vi "ConvertArrayToMessages.vi"(8 "error in (no error)":errorcluster, 11 "Array":bool[][](array[boolean])=array64x128[8192 elements]) -> (0 "error out":errorcluster, 3 "Messages":string[](array[string]))   [LabVIEW 2020, in "CTI-Peripheral.lvlib" / "48x64 I2C OLED SSD1306.lvclass"]
uses:
  48x64 I2C OLED SSD1306.lvclass
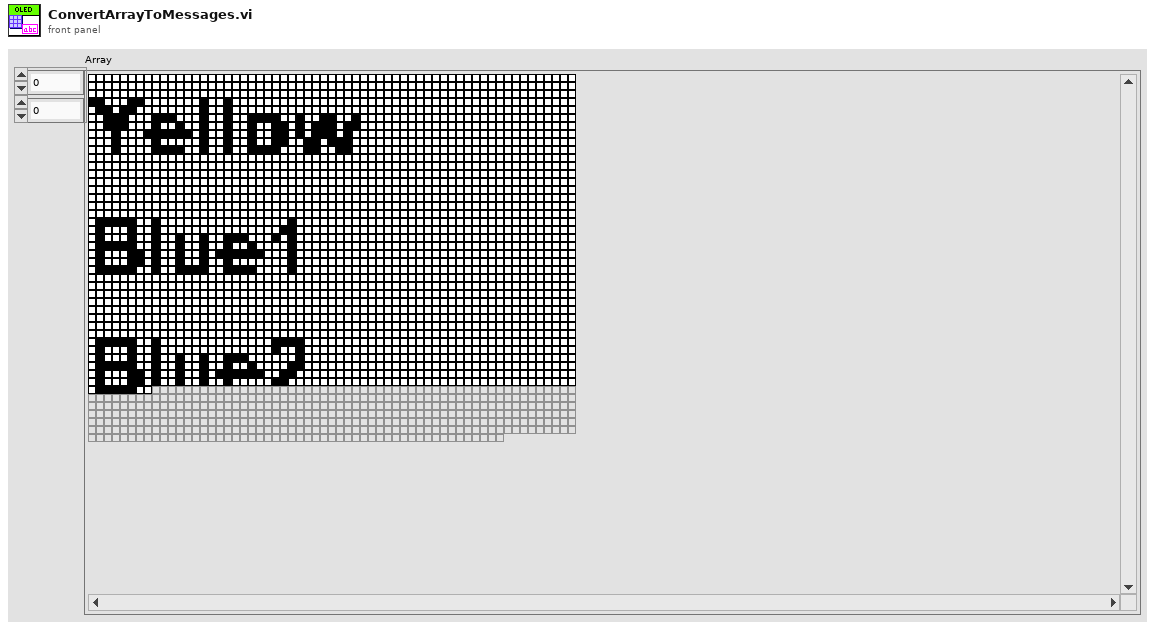
[diagram p1: front panel]
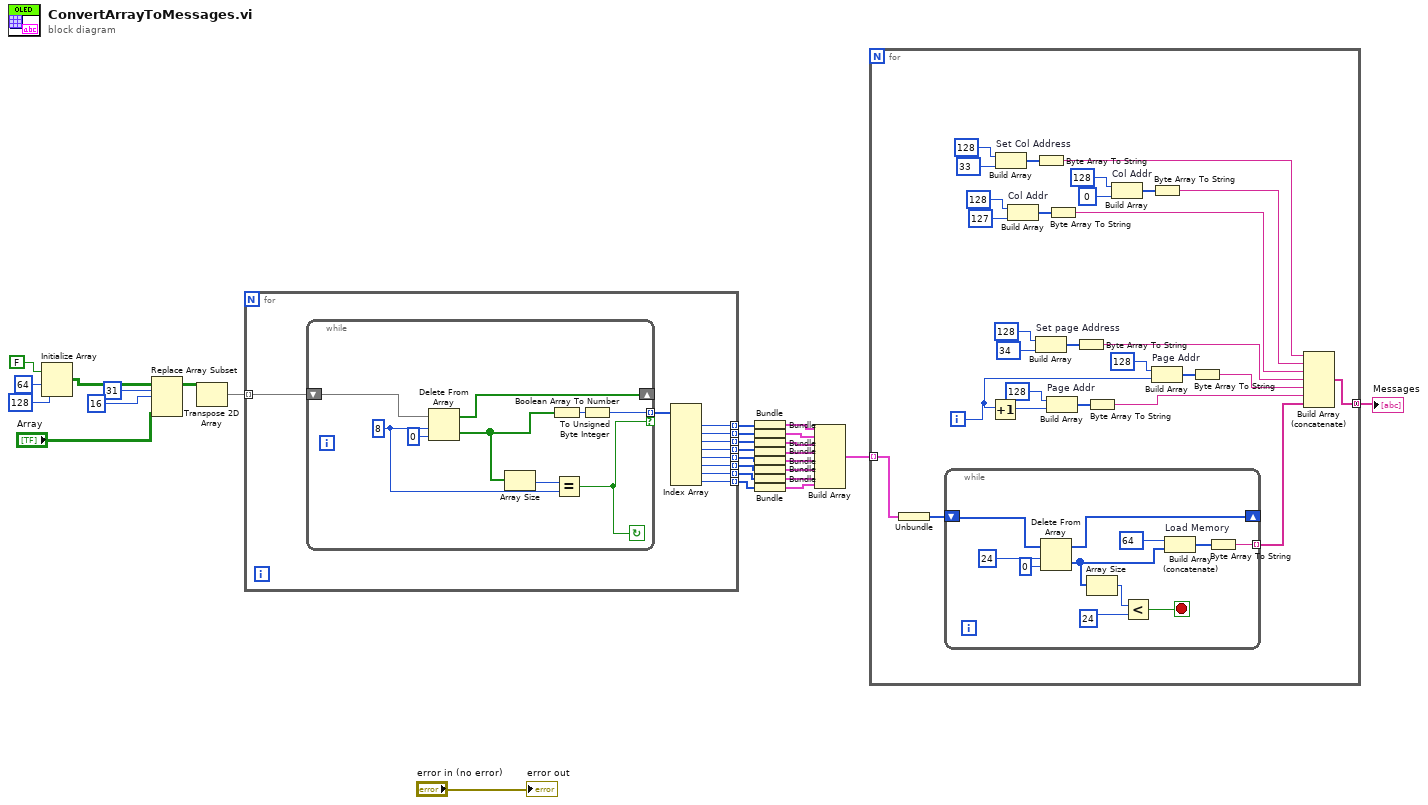
[diagram p0: block diagram]
diagram:
  n1 = Initialize Array(FALSE, 64 ("dimension size"), 128 ("dimension size")) -> (w5:bool[][])
  n2 = Replace Array Subset(array=w5, new element="Array", index (row)=16, index (col)=31 ("disabled index (col)")) -> (w1:bool[][])
  n3 = Transpose 2D Array(2D array=w1) -> (transposed array=w28:bool[][])
  n4 = for {
    tunnel: w28 -> [w29] mode=indexing
    tunnel: [w37] -> w27 mode=indexing
    tunnel: [w36] -> w26 mode=indexing
    tunnel: [w35] -> w25 mode=indexing
    tunnel: [w34] -> w24 mode=indexing
    tunnel: [w33] -> w23 mode=indexing
    tunnel: [w32] -> w22 mode=indexing
    tunnel: [w31] -> w21 mode=indexing
    tunnel: [w30] -> w20 mode=indexing
    n5 = while {
      shift-right: [w43] -> _
      shift-left: w29 -> [w44]
      tunnel: [w47] -> w38 mode=indexing if=w39
      stop <- w39 continue-if-true
      w40 = 8 ("y")
      n6 = Delete From Array(array=w44, length=w40, index=0) -> (deleted portion=w42:bool[], array with subset deleted=w43:bool[])
      n7 = Array Size(array=w42) -> (size(s)=w41:i32)
      n8 = Boolean Array To Number(Boolean array=w42) -> (number=w46:u32)
      n9 = Equal?(x=w41, y=w40) -> (x = y?=w39:bool)
      n10 = To Unsigned Byte Integer(number=w46) -> (unsigned 8bit integer=w47:u8)
    }
    n11 = Index Array(array=w38) -> (element #1=w37:u8, element #2=w36:u8, element #3=w35:u8, element #4=w34:u8, element #5=w33:u8, element #6=w32:u8, element #7=w31:u8, element #8=w30:u8)  [unwired: 8 in]
  }
  n12 = Bundle(w27) -> (w19:cluster{u8[]})  [unwired: 1 in]
  n13 = Bundle(w26) -> (w18:cluster{u8[]})  [unwired: 1 in]
  n14 = Bundle(w25) -> (w17:cluster{u8[]})  [unwired: 1 in]
  n15 = Bundle(w24) -> (w16:cluster{u8[]})  [unwired: 1 in]
  n16 = Bundle(w23) -> (w15:cluster{u8[]})  [unwired: 1 in]
  n17 = Bundle(w22) -> (w14:cluster{u8[]})  [unwired: 1 in]
  n18 = Bundle(w21) -> (w13:cluster{u8[]})  [unwired: 1 in]
  n19 = Bundle(w20) -> (w12:cluster{u8[]})  [unwired: 1 in]
  n20 = Build Array(w19, w18, w17, w16, w15, w14, w13, w12) -> (w10:cluster{u8[]}[])
  n21 = for {
    tunnel: [w75] -> w11 mode=concatenating
    tunnel: w10 -> [w74] mode=indexing
    i -> [w63]
    n22 = Unbundle(w74) -> (w73:u8[])
    n23 = while {
      shift-right: [w83] -> _
      shift-left: w73 -> [w85]
      tunnel: [w77] -> w72 mode=indexing
      stop <- w79 stop-if-true
      n24 = Delete From Array(array=w85, length=24 ("y"), index=0) -> (deleted portion=w81:u8[], array with subset deleted=w83:u8[])
      n25 = Array Size(array=w81) -> (size(s)=w80:i32)
      n26 = Less?(x=w80, y=24) -> (x < y?=w79:bool)
      n27 = Build Array (concatenate) "Load Memory"(u8 64 ("element"), w81) -> (w78:u8[])
      n28 = Byte Array To String(unsigned byte array=w78) -> (string=w77:string)
    }
    n29 = Increment(x=w63) -> (x+1=w64:i32)
    n30 = Build Array "Set Col Address"(u8 128 ("element"), u8 33 ("element")) -> (w57:u8[])
    n31 = Build Array "Col Addr"(u8 128 ("element"), u8 127 ("element")) -> (w51:u8[])
    n32 = Byte Array To String(unsigned byte array=w57) -> (string=w48:string)
    n33 = Build Array "Set page Address"(u8 128 ("element"), u8 34 ("element")) -> (w69:u8[])
    n34 = Build Array "Page Addr"(u8 128 ("element"), w64) -> (w65:i32[])
    n35 = Byte Array To String(unsigned byte array=w51) -> (string=w50:string)
    n36 = Byte Array To String(unsigned byte array=w69) -> (string=w62:string)
    n37 = Byte Array To String(unsigned byte array=w65) -> (string=w60:string)
    n38 = Build Array "Col Addr"(u8 128 ("element"), u8 0 ("element")) -> (w56:u8[])
    n39 = Byte Array To String(unsigned byte array=w56) -> (string=w49:string)
    n40 = Build Array "Page Addr"(u8 128 ("element"), w63) -> (w68:i32[])
    n41 = Byte Array To String(unsigned byte array=w68) -> (string=w61:string)
    n42 = Build Array (concatenate)(w48, w49, w50, w62, w61, w60, w72) -> (w75:string[])
  }
  "Messages" <- w11
  "error out" <- "error in (no error)"
